vi "W5Q1.vi"   [LabVIEW 2021]
uses:
  <vilib>/LabVIEW Interface for Arduino/LabVIEW Interface for Arduino.lvlib
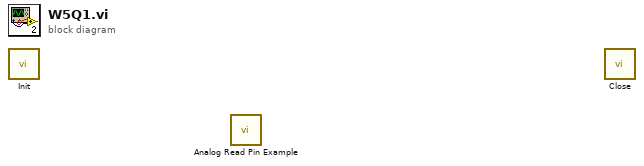
[diagram p0: block diagram]
diagram:
  n1 = call <vilib>:"Init.vi"() -> ()  [unwired: 18 in, 2 out]
  n2 = call <vilib>:"Analog Read Pin Example.vi"() -> ()  [unwired: 12 in]
  n3 = call <vilib>:"Close.vi"() -> ()  [unwired: 15 in, 1 out]
